vi "Test_ethernet_speed.vi"() -> ()   [LabVIEW 2018]
panel:
  out "time elapsed":dbl
  out "error out":errorcluster
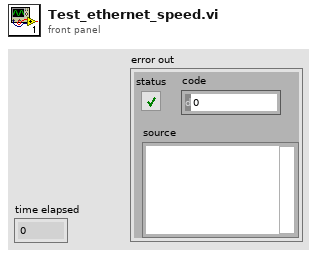
[diagram p1: front panel]
types:
  T1 = enum16{"open", "replace", "create", "open or create", "replace or create", "replace or create with confirmation"}
  T2 = enum16{"big-endian, network order", "native, host order", "little-endian"}
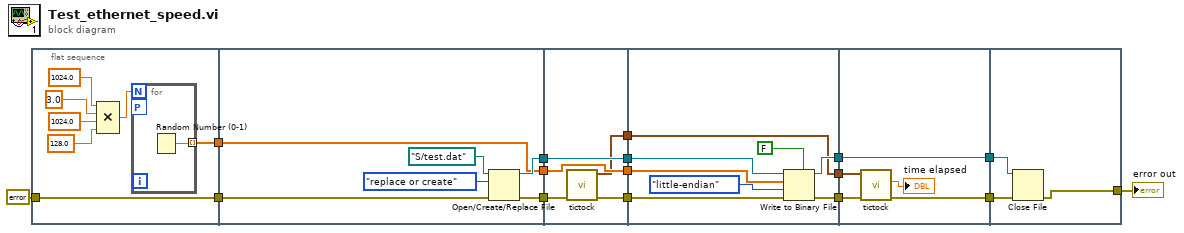
[diagram p0: block diagram]
diagram:
  n1 = flat-sequence {
    tunnel: errorcluster {"status"=FALSE, "code"=0, "source"=""} ("error in") -> [w23]
    tunnel: [w23] -> w15
    tunnel: [w17] -> w14
    tunnel: [w28] -> w13
    tunnel: [w27] -> w12
    tunnel: w15 -> [w29]
    tunnel: [w25] -> w10
    tunnel: w14 -> [w25]
    tunnel: w13 -> [w33]
    tunnel: w12 -> [w35]
    tunnel: [w35] -> w11
    tunnel: w10 -> [w34]
    tunnel: [w34] -> w9
    tunnel: [w32] -> w4
    tunnel: [w31] -> w2
    tunnel: w11 -> [w42]
    tunnel: [w40] -> w8
    tunnel: [w39] -> w6
    tunnel: w9 -> [w37]
    tunnel: w4 -> [w43]
    tunnel: [w36] -> w3
    tunnel: w2 -> [w36]
    tunnel: w8 -> [w47]
    tunnel: [w46] -> w7
    tunnel: w6 -> [w48]
    tunnel: [w48] -> w5
    tunnel: w3 -> [w45]
    tunnel: w7 -> [w51]
    tunnel: w5 -> [w50]
    tunnel: [w49] -> w1
    frame #0 {
      n2 = Compound Arithmetic op=MULTIPLY(1024.0, 3.0, 1024.0, 128.0) -> (w22:dbl)
      n3 = for {
        N: w22 -> [_]
        tunnel: [w24] -> w17 mode=indexing
        workers-P: _ -> [_]
        n4 = Random Number (0-1)() -> (number: 0 to 1=w24:dbl)
      }
    }
    frame #1 {
      n5 = Open/Create/Replace File(file path (use dialog)=path "S:/test.dat", error in=w29, operation (0:open)=T1."replace or create") -> (refnum out=w27:refnum<file>, error out=w28:errorcluster)  [unwired: 3 in, 1 out]
    }
    frame #2 {
      n6 = call "tictock.vi"("error in (no error)"=w33) -> ("error out"=w32:errorcluster, "seconds since 1Jan1904"=w31:timestamp)  [unwired: 8 in, 1 out]
    }
    frame #3 {
      n7 = Write to Binary File(file (use dialog)=w42, data=w37, error in=w43, 5:FALSE ("prepend array or string size? (T)"), 9:T2."little-endian" ("byte order (0:big-endian, network order)")) -> (refnum out=w39:refnum<file>, error out=w40:errorcluster)  [unwired: 1 in, 1 out]
    }
    frame #4 {
      n8 = call "tictock.vi"("error in (no error)"=w47, "seconds since 1Jan1904 2"=w45) -> ("error out"=w46:errorcluster, "Numeric"=→"time elapsed":dbl)  [unwired: 7 in, 1 out]
    }
    frame #5 {
      n9 = Close File(refnum=w50, error in=w51) -> (error out=w49:errorcluster)  [unwired: 1 out]
    }
  }
  "error out" <- w1
